vi "Set Exp Param.vi"(0 "Control-Client in":refnum<class "Control-Client.lvclass">, 11 "error in (no error)":errorcluster) -> (4 "Control-Client out":refnum<class "Control-Client.lvclass">, 15 "error out":errorcluster)   [LabVIEW 2018, in "Control-Client.lvclass"]
uses:
  Control-Client.lvclass
  Control-Client.lvclass/Control-Client.ctl
  Experiments/Experiment.lvclass
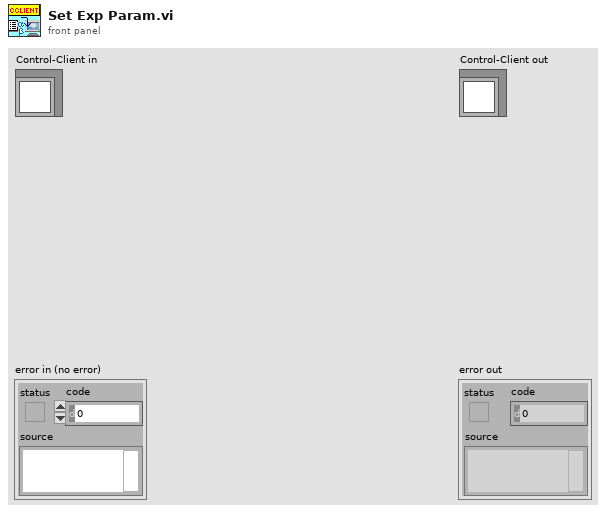
[diagram p1: front panel]
types:
  T1 = typedef "Control-Client.lvclass/Delays-refs_CLIENT.ctl" = cluster{"# points":refnum<vi>, "Step, ps":refnum<vi>, "OZ, ps":refnum<vi>, "# current":refnum<vi>, "RDT, ps":refnum<vi>, "Total length, ps":refnum<vi>, "Kinetics length, ps":refnum<vi>, "Real zero, ps":refnum<vi>, "# par point":refnum<vi>}
  T2 = cluster{"min I, mm":dbl, "max I, mm":dbl, "Real Optical 0, ps":dbl, "min II, mm":dbl, "max II, mm ":dbl}
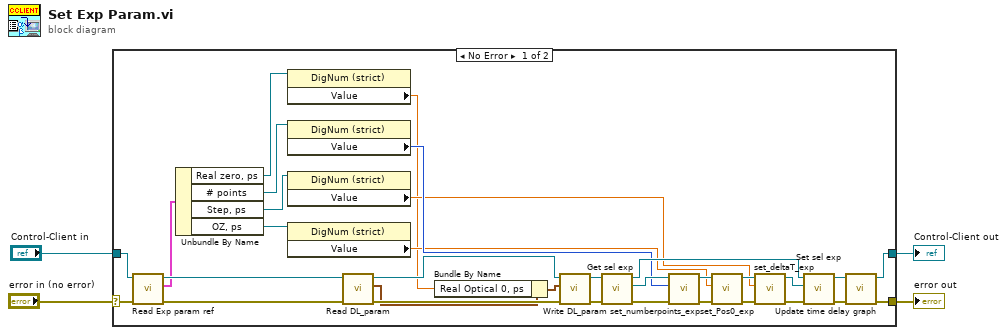
[diagram p0: block diagram]
diagram:
  n1 = case shown="No Error" "error in (no error)" {
    selector: "error in (no error)" -> [w34 w38]
    tunnel: [w10 w38] -> w3
    tunnel: [w11 w37] -> w1
    tunnel: "Control-Client in" -> [w36 w37]
    frame No Error {
      n2 = call "Read Exp param ref.vi"("error in (no error)"=w34, "Control-Client in"=w36) -> ("error out"=w33:errorcluster, "Exp param ref"=w32:T1, "Control-Client out"=w35:refnum<class "Control-Client.lvclass">)  [unwired: 7 in]
      n3 = Unbundle By Name(w32) -> ("Real zero, ps"=w31:refnum<vi>, "# points"=w28:refnum<vi>, "Step, ps"=w29:refnum<vi>, "OZ, ps"=w30:refnum<vi>)
      n4 = property class="DigNum (strict)"(reference=w31) -> ("Value"=w9:dbl)  [unwired: 1 in, 2 out]
      n5 = property class="DigNum (strict)"(reference=w28) -> ("Value"=w14:i32)  [unwired: 1 in, 2 out]
      n6 = property class="DigNum (strict)"(reference=w29) -> ("Value"=w13:dbl)  [unwired: 1 in, 2 out]
      n7 = property class="DigNum (strict)"(reference=w30) -> ("Value"=w12:dbl)  [unwired: 1 in, 2 out]
      n8 = call "Read DL_param.vi"("error in (no error)"=w33, "Control-Client in"=w35) -> ("error out"=w26:errorcluster, "DL_param"=w25:T2, "Control-Client out"=w27:refnum<class "Control-Client.lvclass">)  [unwired: 7 in]
      n9 = Bundle By Name(cluster=w25, "Real Optical 0, ps"=w9) -> (w24:T2)
      n10 = call "Write DL_param.vi"("error in (no error)"=w26, "DL_param"=w24, "Control-Client in"=w27) -> ("error out"=w23:errorcluster, "Control-Client out"=w21:refnum<class "Control-Client.lvclass">)  [unwired: 7 in]
      n11 = call "Get sel exp.vi"("error in (no error)"=w23, "Control-Client in"=w21) -> ("error out"=w19:errorcluster, "Sel experiment"=w20:refnum<class "Experiment.lvclass">, "Control-Client out"=w22:refnum<class "Control-Client.lvclass">)  [unwired: 7 in]
      n12 = call "set_numberpoints_exp.vi"("error in (no error)"=w19, "numberpoints"=w14, "Experiment.lvclass in"=w20) -> ("error out"=w18:errorcluster, "Experiment.lvclass out"=w15:refnum<class "Experiment.lvclass">)  [unwired: 6 in]
      n13 = call "set_Pos0_exp.vi"("error in (no error)"=w18, "Pos0,ps"=w12, "Experiment.lvclass in"=w15) -> ("error out"=w17:errorcluster, "Experiment.lvclass out"=w16:refnum<class "Experiment.lvclass">)  [unwired: 6 in]
      n14 = call "set_deltaT_exp.vi"("error in (no error)"=w17, "deltaTlast"=w13, "Experiment.lvclass in"=w16) -> ("error out"=w8:errorcluster, "Experiment.lvclass out"=w7:refnum<class "Experiment.lvclass">)  [unwired: 6 in]
      n15 = call "Set sel exp.vi"("error in (no error)"=w8, "Experiment"=w7, "Control-Client in"=w22) -> ("error out"=w5:errorcluster, "Control-Client out"=w6:refnum<class "Control-Client.lvclass">)  [unwired: 7 in]
      n16 = call "Update time delay graph.vi"("error in (no error)"=w5, "Control-Client en entrée"=w6) -> ("error out"=w10:errorcluster, "Control-Client en sortie"=w11:refnum<class "Control-Client.lvclass">)  [unwired: 8 in]
    }
    frame Error {
    }
  }
  "error out" <- w3
  "Control-Client out" <- w1
